vi "Set Calibration Data.vi"(0 "Level in":refnum<class "Level.lvclass">, 5 "Freq (Hz)":dbl[](array[numeric]), 7 "Magnitude (dB)":dbl[](array[numeric]), 9 "Phase (degrees)":dbl[](array[numeric]), 11 "error in (no error)":errorcluster) -> (4 "Level out":refnum<class "Level.lvclass">, 15 "error out":errorcluster)   [LabVIEW 2015, in "Level.lvclass"]
uses:
  Level.lvclass
  Level.lvclass/Level.ctl
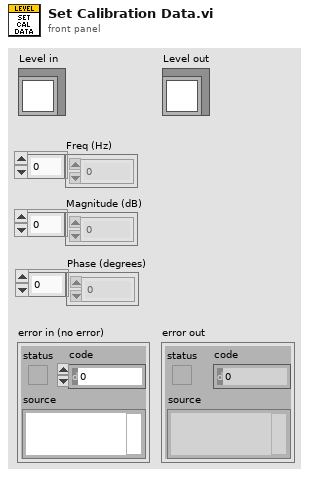
[diagram p1: front panel]
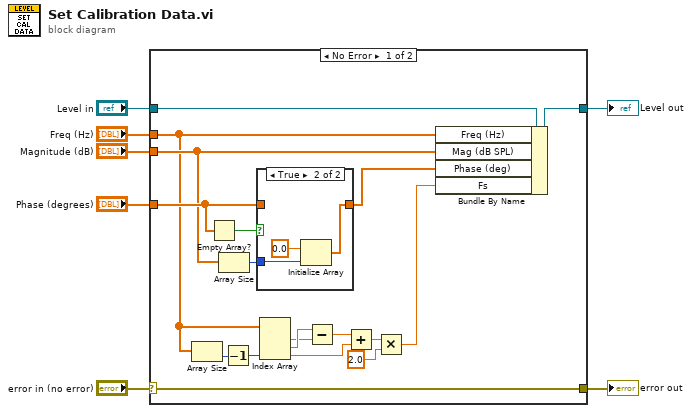
[diagram p0: block diagram]
diagram:
  n1 = case shown="No Error" "error in (no error)" {
    selector: "error in (no error)" -> [w24 w31]
    tunnel: [w24 w31] -> w6
    tunnel: [w23 w30] -> w4
    tunnel: "Level in" -> [w25 w30]
    tunnel: "Freq (Hz)" -> [w15 _]
    tunnel: "Magnitude (dB)" -> [w19 _]
    tunnel: "Phase (degrees)" -> [w20 _]
    frame No Error {
      n2 = Array Size(array=w15) -> (size(s)=w13:i32)
      n3 = Empty Array?(array=w20) -> (empty?=w22:bool)
      n4 = Array Size(array=w19) -> (size(s)=w18:i32)
      n5 = Decrement(x=w13) -> (x-1=w14:i32)
      n6 = case shown="True" w22 {
        tunnel: [w26 w27] -> w21
        tunnel: w20 -> [w26 _]
        tunnel: w18 -> [_ w29]
        frame False {
        }
        frame True {
          n7 = Initialize Array(0.0, w29) -> (w27:dbl[])
        }
      }
      n8 = Index Array(array=w15, index #3=w14) -> (element #1=w16:dbl, element #2=w17:dbl, element #3=w11:dbl)  [unwired: 2 in]
      n9 = Subtract(x=w17, y=w16) -> (x-y=w12:dbl)
      n10 = Add(x=w12, y=w11) -> (x+y=w10:dbl)
      n11 = Multiply(x=w10, y=2.0) -> (x*y=w8:dbl)
      n12 = Bundle By Name(cluster=w25, "Freq (Hz)"=w15, "Mag (dB SPL)"=w19, "Phase (deg)"=w21, "Fs"=w8) -> (w23:refnum<class "Level.lvclass">)
    }
    frame Error {
    }
  }
  "error out" <- w6
  "Level out" <- w4
